vi "Main.vi"(8 "error in (no error)":errorcluster, 10 "Temperature_Notifier":refnum<notifier>, 11 "Message Queues":T1) -> (0 "error out":errorcluster)   [LabVIEW 2019, in "Data_Logger.lvlib"]
uses:
  Data_Logger.lvlib
  Framework/Message Queue/All Message Queues.ctl
  Framework/Message Queue/Message Cluster.ctl
  Logger_Data.ctl
  <vilib>/Utility/sysdir.llb/System Directory Type.ctl
  Framework/Message Queue/Enqueue Message (Single).vi
  Framework/Message Queue/Message Queue.lvlib
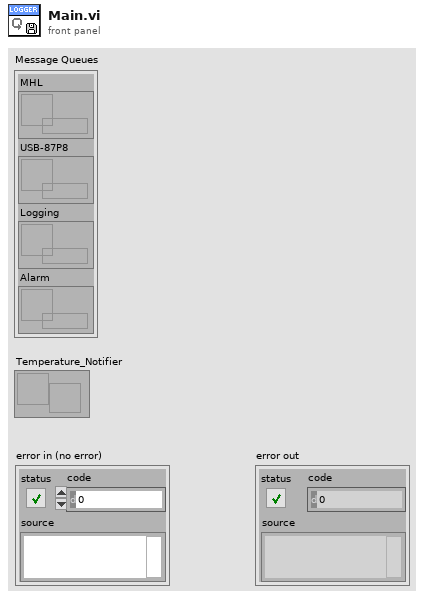
[diagram p1: front panel]
types:
  T1 = typedef "Message Queue.lvlib/All Message Queues.ctl" = cluster{"MHL":refnum<queue>, "USB-87P8":refnum<queue>, "Logging":refnum<queue>, "Alarm":refnum<queue>}
  T2 = typedef "Data_Logger.lvlib/Logger_Data.ctl" = cluster{"Data_Base_Path":path, "Log_File_Ref":refnum<file>, "Timer_Flag":bool, "Log_Interval":dbl, "Config_Base_Path":path}
  T3 = typedef "System Directory Type.ctl" = i32
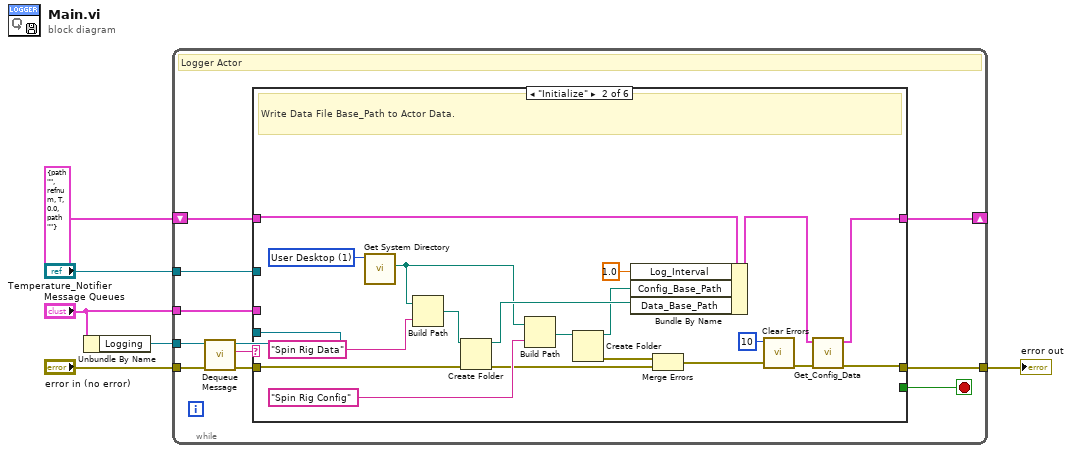
[diagram p0: block diagram]
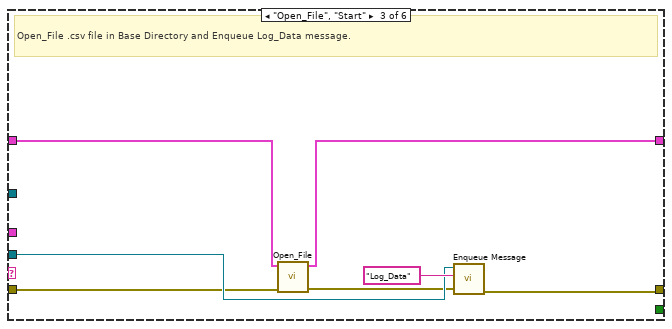
[diagram p3: hidden frame]
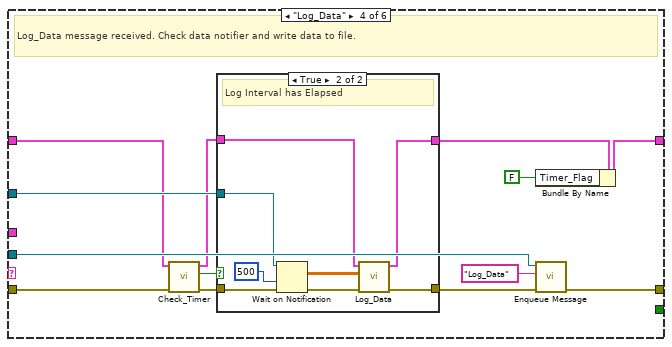
[diagram p4: hidden frame]
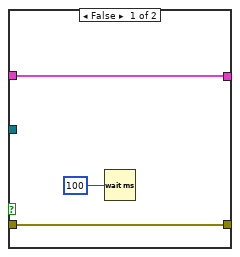
[diagram p5: hidden frame]
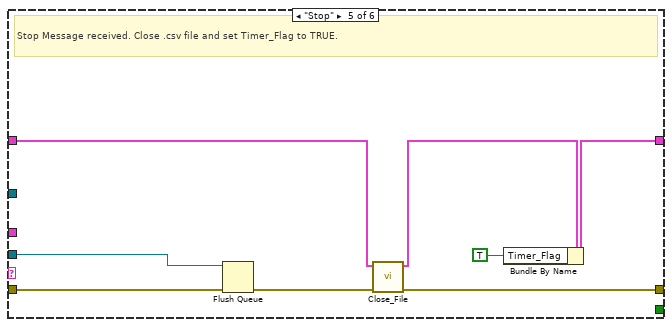
[diagram p6: hidden frame]
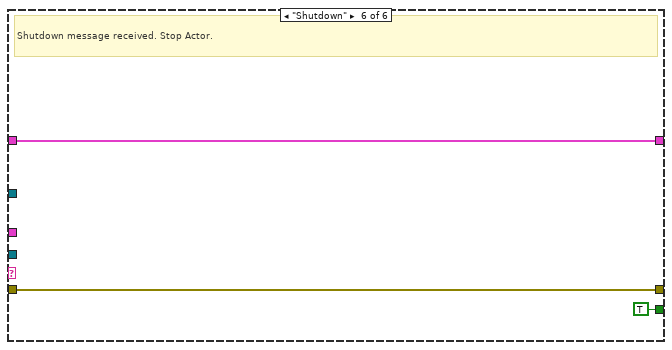
[diagram p7: hidden frame]
diagram:
  n1 = Unbundle By Name("Message Queues") -> ("Logging"=w3:refnum<queue>)
  n2 = while {
    tunnel: "error in (no error)" -> [w17]
    tunnel: "Message Queues" -> [w12]
    tunnel: w3 -> [w16]
    tunnel: [w11] -> w5
    tunnel: "Temperature_Notifier" -> [w9]
    shift-right: [w7] -> _
    shift-left: T2 {"Data_Base_Path"=path "", "Log_File_Ref"=refnum, "Timer_Flag"=TRUE, "Log_Interval"=0.0, "Config_Base_Path"=path ""} -> [w8]
    stop <- w10 stop-if-true
    # "Logger Actor"
    n3 = call "Dequeue Message.vi"("error in (no error)"=w17, "Message Queue"=w16) -> ("error out"=w13:errorcluster, "Message"=w14:string, "dup Message Queue"=w15:refnum<queue>)  [unwired: 6 in, 1 out]
    n4 = case shown="\"Initialize\"" w14 {
      tunnel: w15 -> [_ _ w43 w56 w77 _]
      tunnel: w13 -> [w19 w36 w42 w50 w76 w80]
      tunnel: w12 -> [_ _ _ _ _ _]
      tunnel: [w19 w31 w44 w57 w70 w80] -> w11
      tunnel: [_ _ _ _ _ TRUE] -> w10
      tunnel: w9 -> [_ _ _ w58 _ _]
      tunnel: w8 -> [w18 w38 w41 w48 w72 w78]
      tunnel: [w18 w29 w39 w52 w75 w78] -> w7
      frame Default {
      }
      frame "Initialize" {
        w37 = T3 1 items=["User Home"=0, "User Desktop"=1, "User Documents"=2, "User Application Data"=3, "User Preferences"=4, "User Temporary"=5, "Public Documents"=6, "Public Application Data"=7, "Public Preferences"=8, "Public Cache"=13, "System Core Libraries"=9, "System Installed Libraries"=10, "Application Files"=11, "Boot Volume Root"=12] ("system directory type")
        # "Write Data File Base_Path to Actor Data."
        n5 = call <vilib>:"Get System Directory.vi"("system directory type"=w37) -> ("system directory"=w20:path)  [unwired: 10 in]
        n6 = Build Path(base path=w20, name or relative path="Spin Rig Data") -> (appended path=w28:path)
        n7 = Create Folder(path (use dialog)=w28, error in=w36) -> (created path=w27:path, error out=w22:errorcluster)  [unwired: 1 in, 1 out]
        n8 = Build Path(base path=w20, name or relative path="Spin Rig Config") -> (appended path=w25:path)
        n9 = Create Folder(path (use dialog)=w25) -> (created path=w24:path, error out=w23:errorcluster)  [unwired: 2 in, 1 out]
        n10 = Bundle By Name(cluster=w38, "Log_Interval"=1.0, "Config_Base_Path"=w24, "Data_Base_Path"=w27) -> (w30:T2)
        n11 = Merge Errors(w23, w22) -> (w21:errorcluster)
        n12 = call <vilib>:"Clear Errors.vi"("error in (no error)"=w21, "specific error code to clear (0: all)"=10) -> ("error out"=w32:errorcluster)  [unwired: 4 in, 1 out]
        n13 = call "Get_Config_Data.vi"("error in (no error)"=w32, "Logger_Data In"=w30) -> ("error out"=w31:errorcluster, "Logger_Data Out"=w29:T2)  [unwired: 8 in]
      }
      frame "Open_File", "Start" {
        # "Open_File .csv file in Base Directory and Enqueue Log_Data message."
        n14 = call "Open_File.vi"("error in (no error)"=w42, "Logger_Data In"=w41) -> ("error out"=w40:errorcluster, "Logger_Data Out"=w39:T2)  [unwired: 8 in]
        n15 = call-poly "Enqueue Message.vi"("error in (no error)"=w40, "Message"="Log_Data", "Message Queue"=w43) -> ("error out"=w44:errorcluster)  [unwired: 7 in, 1 out]
      }
      frame "Log_Data" {
        # "Log_Data message received. Check data notifier and write data to file."
        n16 = call "Check_Timer.vi"("error in (no error)"=w50, "Logger_Data In"=w48) -> ("error out"=w49:errorcluster, "Time has Elapsed"=w46:bool, "Logger_Data Out"=w47:T2)  [unwired: 7 in]
        n17 = case shown="True" w46 {
          tunnel: w58 -> [_ w69]
          tunnel: [w60 w65] -> w54
          tunnel: [w61 w64] -> w53
          tunnel: w49 -> [w60 w63]
          tunnel: w47 -> [w61 w62]
          frame False {
            n18 = Wait (ms)(milliseconds to wait=u32 100) -> ()  [unwired: 1 out]
          }
          frame True {
            # "Log Interval has Elapsed"
            n19 = Wait on Notification(notifier=w69, timeout in ms (-1)=500, error in (no error)=w63) -> (notification=w67:sgl[][], error out=w66:errorcluster)  [unwired: 1 in, 2 out]
            n20 = call "Log_Data.vi"("error in (no error)"=w66, "Data"=w67, "Logger_Data In"=w62) -> ("error out"=w65:errorcluster, "Logger_Data Out"=w64:T2)  [unwired: 7 in]
          }
        }
        n21 = Bundle By Name(cluster=w53, "Timer_Flag"=FALSE) -> (w52:T2)
        n22 = call-poly "Enqueue Message.vi"("error in (no error)"=w54, "Message"="Log_Data", "Message Queue"=w56) -> ("error out"=w57:errorcluster)  [unwired: 7 in, 1 out]
      }
      frame "Stop" {
        # "Stop Message received. Close .csv file and set Timer_Flag to TRUE."
        n23 = Flush Queue(queue=w77, error in (no error)=w76) -> (error out=w73:errorcluster)  [unwired: 2 out]
        n24 = call "Close_File.vi"("error in (no error)"=w73, "Log_Data In"=w72) -> ("error out"=w70:errorcluster, "Log_Data Out"=w71:T2)  [unwired: 8 in]
        n25 = Bundle By Name(cluster=w71, "Timer_Flag"=TRUE) -> (w75:T2)
      }
      frame "Shutdown" {
        # "Shutdown message received. Stop Actor."
      }
    }
  }
  "error out" <- w5
